vi "Arm Controller.vi"(8 "error in":errorcluster) -> ()   [LabVIEW 2019]
doc: "This VI executes continuously carrying out the current operation and responding to updates or new operations. It will often contain the timing or control code that is difficult to place directly in TeleOp. This VI generally opens all sensors and motors and isolates the rest of the robot code from knowing how the operations are carried out."
uses:
  <vilib>/Rock Robotics/WPI/Framework/Completion Status.ctl
  Arm Setpoints.ctl
  Arm Operations.ctl
  <vilib>/Rock Robotics/WPI/SafetyOutput/WPI_SafetyOutputConfigMenu.ctl
  <vilib>/Rock Robotics/SystemInterfaces/DIO/FPGA_DIOChannel.ctl
  <vilib>/Rock Robotics/WPI/Counter/WPI_CounterDigitalInputToDigitalSource.vi
  <vilib>/Rock Robotics/WPI/Switch/WPI_SwitchOpenLimit.vi
  <vilib>/addons/control/pid/pid.llb/PID (DBL).vi
  <vilib>/Rock Robotics/Network Tables/NT Write Boolean.vi
  <vilib>/addons/control/pid/NI_PID_pid.lvlib
panel:
  in  "Interactive Values":T1
  out "Current\nCmd":string
  in  "Buttons":cluster{"Execute Cmd":bool, "Abort Cmd":bool}
  out "Command Timing":cluster{"Start Time (ms)":u32, "Iterations":i32}
  out "Status":T3
  # "Tip: It may be helpful to observe inputs and sensor values.\nYou may also want to display tuning or debugging controls."
  # "Interactive Command: You may fill in the settings for a command\nand schedule it with the Execute button. You can observe and abort\nany command while fine tuning the code for the controller."
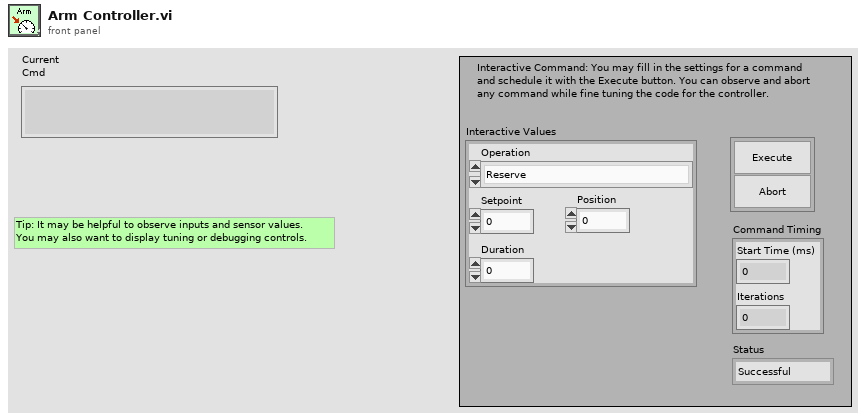
[diagram p1: front panel]
types:
  T1 = typedef "Arm Setpoints.ctl" = cluster{"Operation":T2, "Setpoint":dbl, "Duration":dbl, "Position":dbl}
  T2 = typedef "Arm Operations.ctl" = enum16{"Reserve", "Read Current", "Immediate", "PositionDrive", "ZeroArm"}
  T3 = typedef "Completion Status.ctl" = enum16{"Successful", "Aborted", "Incomplete"}
  T4 = typedef "FPGA_DIOChannel.ctl" = enum8{"DIO 0", "DIO 1", "DIO 2", "DIO 3", "DIO 4", "DIO 5", "DIO 6", "DIO 7", "DIO 8", "DIO 9", "DIO MXP 0", "DIO MXP 1", "DIO MXP 2", "DIO MXP 3", "DIO MXP 4", "DIO MXP 5", "DIO MXP 6", "DIO MXP 7", "DIO MXP 8", "DIO MXP 9", "DIO MXP 10", "DIO MXP 11", "DIO MXP 12", "DIO MXP 13", "DIO MXP 14", "DIO MXP 15", "SPI Port CS1", "SPI Port CS2", "SPI Port CS3", "SPI Port MISO", "SPI Port MOSI", "Invalid"}
  T5 = typedef "WPI_SafetyOutputConfigMenu.ctl" = enum16{"Enable", "Disable"}
  T6 = typedef "WPI_SwitchDevRef.ctl" = cluster{"DevStatus":errorcluster, "DIO Channel":T4, "CntIndex":T7, "Normally Closed":bool}
  T7 = typedef "FPGA_CounterCtrSystemIndex.ctl" = enum8{"Ctr 0", "Ctr 1", "Ctr 2", "Ctr 3", "Ctr 4", "Ctr 5", "Ctr 6", "Ctr 7", "Invalid"}
  T8 = typedef "WPI_MotorControlDeviceRef.ctl" = cluster{"DeviceStatus":errorcluster, "Type":T9, "PWM":cluster{"PWM Channel":T10, "DeadBand":T11}, "CAN":cluster{"Device Number":u8, "SetOutput VI Ref":variant, "GetOutput VI Ref":variant, "Enable VI Ref":variant, "Disable VI Ref":variant, "Data":variant}, "Invert":bool, "DIO PWM":cluster{"PWM \"Enable\" Channel":T10, "DIOChannel":T4, "PWM Rate":dbl}}
  T9 = typedef "WPI_MotorControlType.ctl" = enum16{"PWM", "CAN", "DIO PWM"}
  T10 = typedef "FPGA_DIOPWMChannel.ctl" = enum8{"PWM 0", "PWM 1", "PWM 2", "PWM 3", "PWM 4", "PWM 5", "PWM 6", "PWM 7", "PWM 8", "PWM 9", "PWM MXP 0", "PWM MXP 1", "PWM MXP 2", "PWM MXP 3", "PWM MXP 4", "PWM MXP 5", "PWM MXP 6", "PWM MXP 7", "PWM MXP 8", "PWM MXP 9", "Invalid"}
  T11 = typedef "WPI_PWMDeadband.ctl" = cluster{"Name":string, "maxPositivePwm":i32, "minPositivePwm":i32, "centerPwm":i32, "maxNegativePwm":i32, "minNegativePwm":i32, "angularRange":u16}
  T12 = typedef "WPI_DigitalInputDevRef.ctl" = cluster{"DevStatus":errorcluster, "DIO Channel":T4}
  T13 = typedef "FPGA_CounterEncoderSourceConvertionLVSourceType.ctl" = cluster{"DevStatus":errorcluster, "AnalogTriggerMode?":bool, "DigitalMode":cluster{"DIO Channel":T14}, "AnalogTriggerMode":cluster{"AnalogTriggerIndex":T15, "OutputType":T16}}
  T14 = typedef "FPGA_DIODigitalSourceChannel.ctl" = enum8{"DIO 0", "DIO 1", "DIO 2", "DIO 3", "DIO 4", "DIO 5", "DIO 6", "DIO 7", "DIO 8", "DIO 9", "DIO MXP 0", "DIO MXP 1", "DIO MXP 2", "DIO MXP 3", "DIO MXP 4", "DIO MXP 5", "DIO MXP 6", "DIO MXP 7", "DIO MXP 8", "DIO MXP 9", "DIO MXP 10", "DIO MXP 11", "DIO MXP 12", "DIO MXP 13", "DIO MXP 14", "DIO MXP 15", "SPI Port CS1", "SPI Port CS2", "SPI Port CS3", "SPI Port MISO", "SPI Port MOSI", "Disabled"}
  T15 = typedef "FPGA_AnalogTriggerIndex.ctl" = enum8{"Trig 0", "Trig 1", "Trig 2", "Trig 3", "Trig 4", "Trig 5", "Trig 6", "Trig 7", "Invalid"}
  T16 = typedef "FPGA_AnalogTriggerOutType.ctl" = enum16{"InWindow", "TriggerState", "Rising", "Falling"}
  T17 = typedef "WPI_EncoderDevRef.ctl" = cluster{"DevStatus":errorcluster, "EncoderIndex":T18, "CounterIndex":T7, "DistancePerCount":dbl, "Decoding Type":T19}
  T18 = typedef "FPGA_EncoderIdx.ctl" = enum8{"Enc 0", "Enc 1", "Enc 2", "Enc 3", "Enc 4", "Enc 5", "Enc 6", "Enc 7", "Invalid"}
  T19 = typedef "WPI_EncoderType.ctl" = enum16{"1x", "2x", "4x"}
  T20 = typedef "Command Status Info.ctl" = cluster{"Name":string, "Status":T3, "notifier out":T21}
  T21 = typedef "Completion Notifier.ctl" = refnum<notifier>
  T22 = cluster{"Current Command":T1, "Command Timing":cluster{"Start Time (ms)":u32, "Iterations":i32}, "Command Arguments":cluster{"Command Info":T20, "Description":string, "Default Command":T1, "queue out":refnum<queue>, "Subsystem Name":string}}
  T23 = cluster{"proportional gain (Kc)":dbl, "integral time (Ti, min)":dbl, "derivative time (Td, min)":dbl}
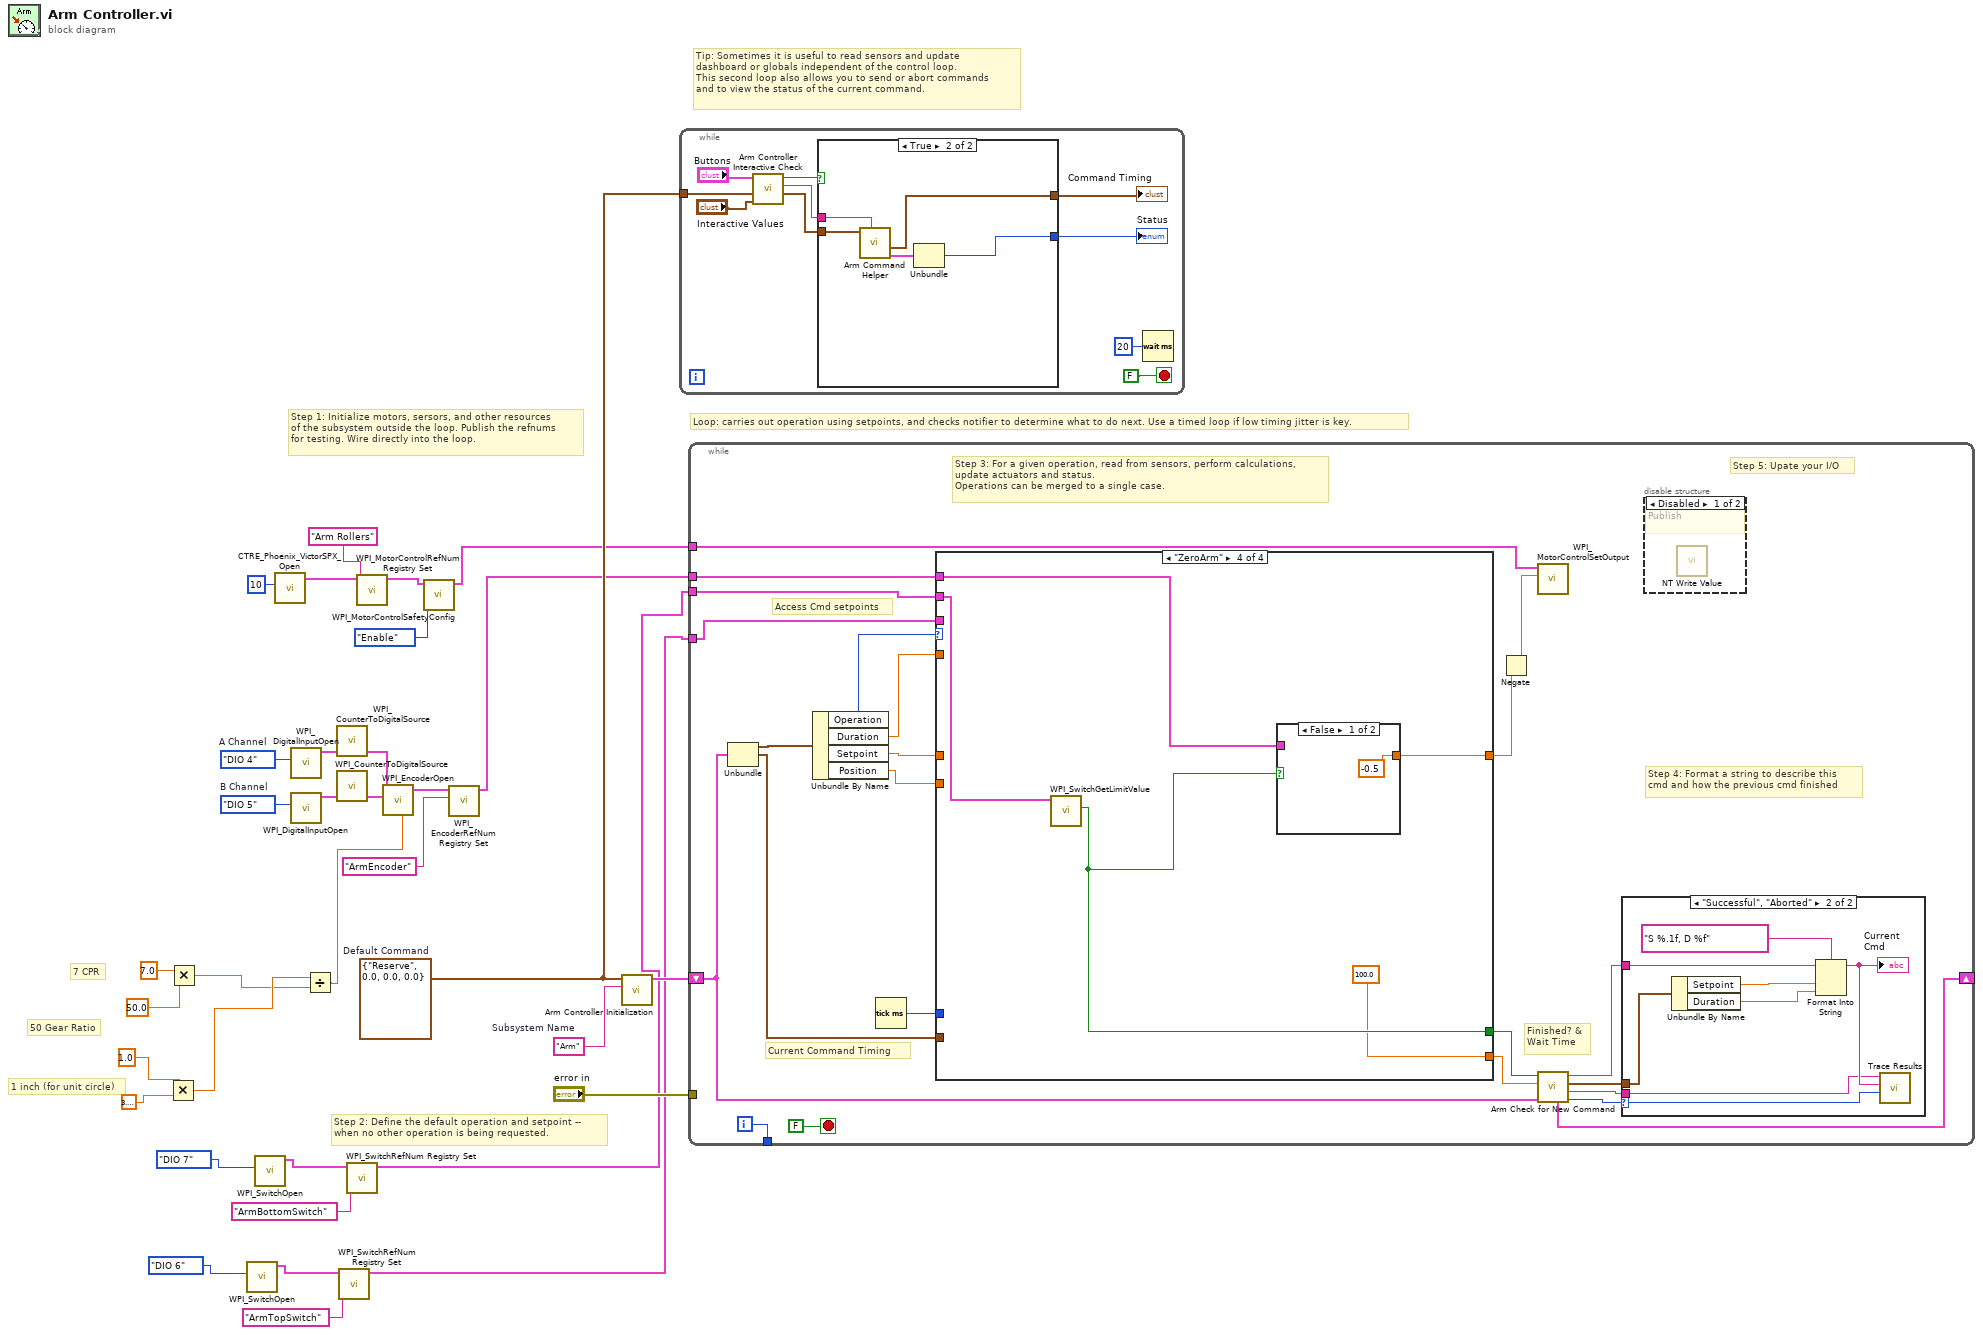
[diagram p0: block diagram]
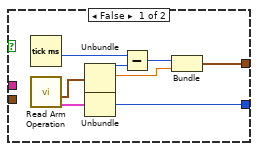
[diagram p2: hidden frame]
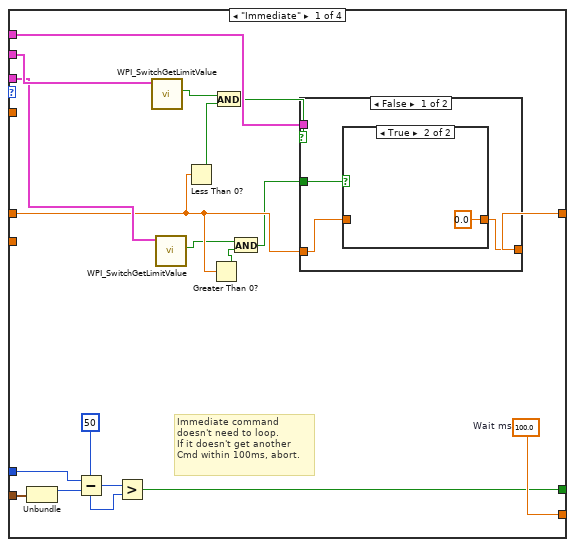
[diagram p5: hidden frame]
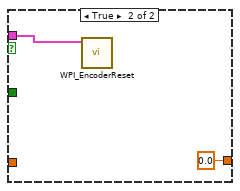
[diagram p7: hidden frame]
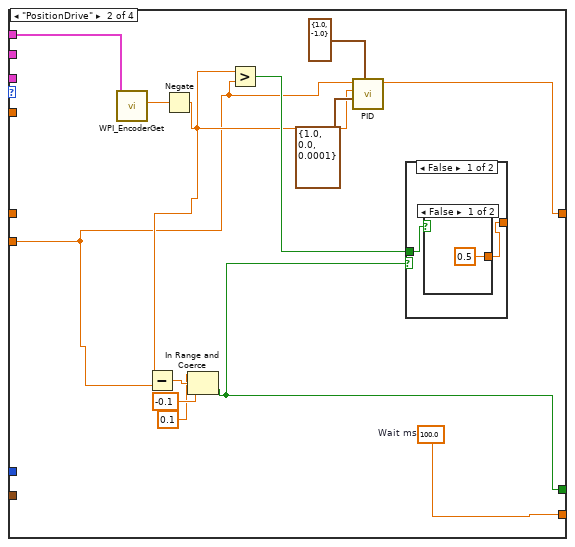
[diagram p8: hidden frame]
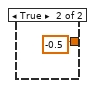
[diagram p9: hidden frame]
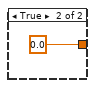
[diagram p10: hidden frame]
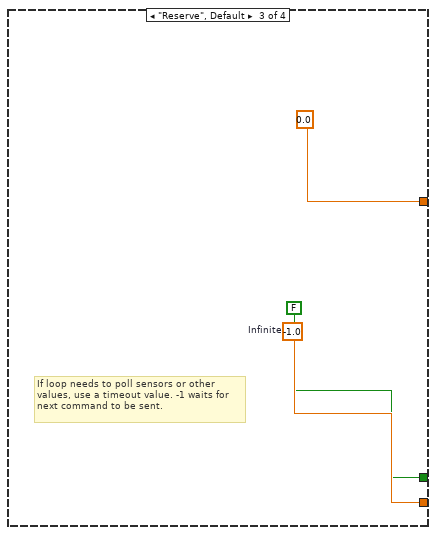
[diagram p11: hidden frame]
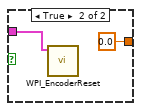
[diagram p12: hidden frame]
diagram:
  w24 = FPGA_DIOChannel."DIO 5"  # B Channel
  w23 = FPGA_DIOChannel."DIO 4"  # A Channel
  w31 = T1 {"Operation"=enum."Reserve", "Setpoint"=0.0, "Duration"=0.0, "Position"=0.0}  # Default Command
  w32 = "Arm"  # Subsystem Name
  # "1 inch (for unit circle)"
  # "50 Gear Ratio"
  # "7 CPR"
  # "Tip: Sometimes it is useful to read sensors and update\ndashboard or globals independent of the control loop.\nThis second loop also allows you to send or abort commands\nand to view the status of the current command."
  # "Step 2: Define the default operation and setpoint --\nwhen no other operation is being requested."
  # "Step 1: Initialize motors, sersors, and other resources\nof the subsystem outside the loop. Publish the refnums\nfor testing. Wire directly into the loop."
  # "Loop: carries out operation using setpoints, and checks notifier to determine what to do next. Use a timed loop if low timing jitter is key."
  n1 = Multiply(x=1.0 ("DistancePerCount"), y=3.141592653589793) -> (x*y=w11:dbl)
  n2 = Multiply(x=7.0, y=50.0) -> (x*y=w10:dbl)
  n3 = call-poly <vilib>:"WPI_SwitchOpen.vi"("DIO Channel"=FPGA_DIOChannel."DIO 6") -> ("SwitchDevRef"=w3:T6)  [unwired: 9 in, 1 out]
  n4 = call-poly <vilib>:"WPI_SwitchOpen.vi"("DIO Channel"=FPGA_DIOChannel."DIO 7") -> ("SwitchDevRef"=w7:T6)  [unwired: 9 in, 1 out]
  n5 = call <vilib>:"CTRE_Phoenix_VictorSPX_Open.vi"("Device Number"=u8 10) -> ("CAN Talon SRX Ref"=w28:T8)  [unwired: 9 in, 1 out]
  n6 = call <vilib>:"WPI_DigitalInputOpen.vi"("DIO Channel"=w23) -> ("DigitalInputDevRef"=w20:T12)  [unwired: 1 in, 9 out]
  n7 = call <vilib>:"WPI_DigitalInputOpen.vi"("DIO Channel"=w24) -> ("DigitalInputDevRef"=w21:T12)  [unwired: 1 in, 9 out]
  n8 = Divide(x=w11, y=w10) -> (x/y=w9:dbl)
  n9 = call-poly <vilib>:"WPI_CounterToDigitalSource.vi"("DigitalInputDevRef"=w20) -> ("Digital Source"=w19:T13)  [unwired: 6 out]
  n10 = call-poly <vilib>:"WPI_CounterToDigitalSource.vi"("DigitalInputDevRef"=w21) -> ("Digital Source"=w22:T13)  [unwired: 6 out]
  n11 = call <vilib>:"WPI_SwitchRefNum Registry Set.vi"("refnum name"="ArmTopSwitch", "SwitchDevRef"=w3) -> ("SwitchDevRef"=w1:T6)  [unwired: 8 in, 1 out]
  n12 = call <vilib>:"WPI_SwitchRefNum Registry Set.vi"("refnum name"="ArmBottomSwitch", "SwitchDevRef"=w7) -> ("SwitchDevRef"=w5:T6)  [unwired: 8 in, 1 out]
  n13 = call <vilib>:"WPI_MotorControlRefNum Registry Set.vi"("refnum name"="Arm Rollers", "MotorControlDevRef"=w28) -> ("MotorControlDevRef"=w29:T8)  [unwired: 8 in, 1 out]
  n14 = call <vilib>:"WPI_EncoderOpen.vi"("DistancePerCount"=w9, "BSource"=w22, "ASource"=w19) -> ("EncoderDevRef"=w18:T17)  [unwired: 5 in, 3 out]
  n15 = call <vilib>:"WPI_MotorControlSafetyConfig.vi"("mode"=WPI_SafetyOutputConfigMenu."Enable", "MotorControlDevRef"=w29) -> ("MotorControlDevRef"=w25:T8)  [unwired: 8 in, 1 out]
  n16 = call <vilib>:"WPI_EncoderRefNum Registry Set.vi"("refnum name"="ArmEncoder", "EncoderDevRef"=w18) -> ("EncoderDevRef"=w16:T17)  [unwired: 8 in, 1 out]
  n17 = call "Arm Controller Initialization.vi"("Subsystem Name"=w32, "Default Command"=w31) -> ("Current Command"=w33:T22)  [unwired: 9 in]
  n18 = while {
    tunnel: w31 -> [w41]
    stop <- FALSE stop-if-true
    n19 = call "Arm Controller Interactive Check.vi"("Interactive Command in"="Interactive Values", "Default Command"=w41, "Buttons"="Buttons") -> ("Interactive Command out"=w38:T1, "Trace String"=w39:string, "Schedule"=w40:bool)  [unwired: 6 in]
    n20 = case shown="True" w40 {
      tunnel: [w52 w57] -> w37
      tunnel: w38 -> [_ w55]
      tunnel: [w48 w53] -> w36
      tunnel: w39 -> [_ w56]
      frame False {
        n21 = Tick Count (ms)() -> (millisecond timer value=w47:u32)
        n22 = call "Read Arm Operation.vi"() -> ("Command Info"=w45:T20, "SubSystem Data"=w46:T1)  [unwired: 9 in, 1 out]
        n23 = Unbundle(w46) -> ("Operation"=w51:T2, "Setpoint"=w49:dbl)  [unwired: 2 out]
        n24 = Unbundle(w45) -> ("Status"=w52:T3)  [unwired: 2 out]
        n25 = Subtract(x=w47, y=w51) -> (x-y=w50:u32)
        n26 = Bundle(w50, "Setpoint"=w49) -> (w48:cluster{u32, "Setpoint":dbl})  [unwired: 1 in]
      }
      frame True {
        n27 = call "Arm Command Helper.vi"("Description"=w56, "SubSystem Data"=w55) -> ("Command Info Out"=w54:T20, "Command Timing"=w53:cluster{"Start Time (ms)":u32, "Iterations":i32})  [unwired: 7 in, 1 out]
        n28 = Unbundle(w54) -> ("Status"=w57:T3)  [unwired: 2 out]
      }
    }
    "Status" <- w37
    "Command Timing" <- w36
    n29 = Wait (ms)(milliseconds to wait=u32 20) -> ()  [unwired: 1 out]
  }
  n30 = while {
    shift-right: [w72] -> _
    shift-left: w33 -> [w65]
    tunnel: [w79] -> _
    tunnel: "error in" -> [_]
    tunnel: w25 -> [w64]
    tunnel: w16 -> [w62]
    tunnel: w5 -> [w60]
    tunnel: w1 -> [w59]
    i -> [w79]
    stop <- FALSE stop-if-true
    # "Step 5: Upate your I/O"
    # "Step 4: Format a string to describe this\ncmd and how the previous cmd finished"
    # "Current Command Timing"
    # "Access Cmd setpoints"
    # "Finished? &\nWait Time"
    # "Step 3: For a given operation, read from sensors, perform calculations,\nupdate actuators and status.\nOperations can be merged to a single case."
    n31 = Unbundle(w65) -> ("Current Command"=w78:T1, "Command Timing"=w74:cluster{"Start Time (ms)":u32, "Iterations":i32})  [unwired: 1 out]
    n32 = Unbundle By Name(w78) -> ("Operation"=w77:T2, "Duration"=w76:dbl, "Setpoint"=w73:dbl, "Position"=w63:dbl)
    n33 = Tick Count (ms)() -> (millisecond timer value=w75:u32)
    n34 = case shown="\"ZeroArm\"" w77 {
      tunnel: [w106 w125 w134 100.0 ("Infinite")] -> w70
      tunnel: [w100 w122 FALSE ("ignore previous (F)") w138] -> w71
      tunnel: w74 -> [w102 _ _ _]
      tunnel: w76 -> [_ _ _ _]
      tunnel: w75 -> [w101 _ _ _]
      tunnel: w73 -> [w92 _ _ _]
      tunnel: [w98 w117 0.0 ("Setpoint") w137] -> w61
      tunnel: w63 -> [_ w115 _ _]
      tunnel: w62 -> [w97 w126 _ w136]
      tunnel: w60 -> [w99 _ _ w139]
      tunnel: w59 -> [w96 _ _ _]
      frame "Immediate" {
        w106 = 100.0  # Wait ms
        # "Immediate command\ndoesn't need to loop.\nIf it doesn't get another\nCmd within 100ms, abort."
        n35 = Unbundle(w102) -> ("Start Time (ms)"=w105:u32)  [unwired: 1 out]
        n36 = Subtract(x=w101, y=w105) -> (x-y=w104:u32)
        n37 = Greater?(x=w104, y=u8 50 ("Left Motor")) -> (0:w100:bool)
        n38 = call <vilib>:"WPI_SwitchGetLimitValue.vi"("SwitchDevRef"=w99) -> ("Switch Pressed"=w93:bool)  [unwired: 8 in, 2 out]
        n39 = call <vilib>:"WPI_SwitchGetLimitValue.vi"("SwitchDevRef"=w96) -> ("Switch Pressed"=w90:bool)  [unwired: 8 in, 2 out]
        n40 = Less Than 0?(x=w92) -> (x < 0?=w94:bool)
        n41 = Greater Than 0?(x=w92) -> (x > 0?=w91:bool)
        n42 = And(x=w93, y=w94) -> (x .and. y?=w95:bool)
        n43 = And(x=w90, y=w91) -> (x .and. y?=w89:bool)
        n44 = case shown="False" w95 {
          tunnel: w92 -> [w108 _]
          tunnel: [w107 0.0 ("Setpoint")] -> w98
          tunnel: w97 -> [_ w112]
          tunnel: w89 -> [w109 _]
          frame False {
            n45 = case shown="True" w109 {
              tunnel: w108 -> [w110 _]
              tunnel: [w110 0.0 ("Setpoint")] -> w107
              frame False {
              }
              frame True {
              }
            }
          }
          frame True {
            n46 = call <vilib>:"WPI_EncoderReset.vi"("EncoderDevRef"=w112) -> ()  [unwired: 9 in, 2 out]
          }
        }
      }
      frame "PositionDrive" {
        w125 = 100.0  # Wait ms
        n47 = call <vilib>:"WPI_EncoderGet.vi"("EncoderDevRef"=w126) -> ("Distance"=w124:dbl)  [unwired: 5 in, 5 out]
        n48 = Negate(x=w124) -> (-x=w116:dbl)
        n49 = Subtract(x=w116, y=w115) -> (x-y=w121:dbl)
        n50 = In Range and Coerce(upper limit=0.1 ("x"), x=w121, lower limit=-0.1) -> (In Range?=w122:bool)  [unwired: 1 out]
        n51 = Greater?(x=w116, y=w115) -> (0:w123:bool)
        n52 = call-poly <vilib>:"PID.vi"("output range"=cluster{"output high":dbl, "output low":dbl} {"output high"=1.0, "output low"=-1.0}, "PID gains"=T23 {"proportional gain (Kc)"=1.0, "integral time (Ti, min)"=0.0, "derivative time (Td, min)"=0.0001}, "process variable"=w116, "setpoint"=w115) -> ("output"=w117:dbl)  [unwired: 6 in, 1 out]
        n53 = case shown="False" w122 {
          tunnel: [w128 0.0] -> _
          tunnel: w123 -> [w127 _]
          frame False {
            n54 = case shown="False" w127 {
              tunnel: [0.5 -0.5] -> w128
              frame False {
              }
              frame True {
              }
            }
          }
          frame True {
          }
        }
      }
      frame "Reserve", Default {
        w134 = -1.0  # Infinite
        # "If loop needs to poll sensors or other\nvalues, use a timeout value. -1 waits for\nnext command to be sent."
      }
      frame "ZeroArm" {
        n55 = call <vilib>:"WPI_SwitchGetLimitValue.vi"("SwitchDevRef"=w139) -> ("Switch Pressed"=w138:bool)  [unwired: 8 in, 2 out]
        n56 = case shown="False" w138 {
          tunnel: [-0.5 0.0] -> w137
          tunnel: w136 -> [_ w141]
          frame False {
          }
          frame True {
            n57 = call <vilib>:"WPI_EncoderReset.vi"("EncoderDevRef"=w141) -> ()  [unwired: 9 in, 2 out]
          }
        }
      }
    }
    n58 = Negate(x=w61) -> (-x=w58:dbl)
    n59 = call <vilib>:"WPI_MotorControlSetOutput.vi"("Output"=w58, "MotorControlDevRef"=w64) -> ()  [unwired: 7 in, 3 out]
    n60 = call "Arm Check for New Command.vi"("Current Command"=w65, "Wait time (ms)"=w70, "Finished?"=w71) -> ("Completion"=w66:T3, "Subsystem Name"=w67:string, "Current Command"=w68:T1, "Initial Trace String"=w69:string, "NextCommand"=w72:T22)  [unwired: 4 in]
    n61 = case shown="\"Successful\", \"Aborted\"" w66 {
      selector: w66 -> [_ w88]
      tunnel: w69 -> [_ w84]
      tunnel: w68 -> [_ w85]
      tunnel: w67 -> [_ w81]
      frame "Incomplete", Default {
        # "Continuing current command"
      }
      frame "Successful", "Aborted" {
        # "Report and setup for next command"
        n62 = Unbundle By Name(w85) -> ("Setpoint"=w87:dbl, "Duration"=w82:dbl)
        n63 = Format Into String(format string="S %.1f, D %f", initial string=w84, w87, w82) -> (resulting string=w83:string)  [unwired: 1 in, 1 out]
        "Current\nCmd" <- w83
        n64 = call <vilib>:"Trace Results.vi"("Status of previous command"=w88, "Description"=w83, "Subsystem"=w81) -> ()  [unwired: 9 in]
      }
    }
    n65 = disable-structure shown="Disabled" {
      frame Disabled {
        # "Publish"
        n66 = call-poly <vilib>:"NT Write Value.vi"() -> ()  [unwired: 11 in, 1 out]
      }
      frame Enabled {
      }
    }
  }
